vi "Stop Test.vi"(8 "ErrorIn":errorcluster, 11 "VISAIn":refnum<visa-resource-name>) -> (0 "ErrorOut":errorcluster, 2 "Data":string, 3 "VISAOut":refnum<visa-resource-name>)   [LabVIEW 2017, in "I28Drivers.lvlib"]
uses:
  I28Drivers.lvlib
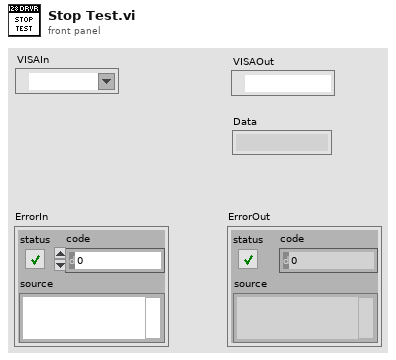
[diagram p1: front panel]
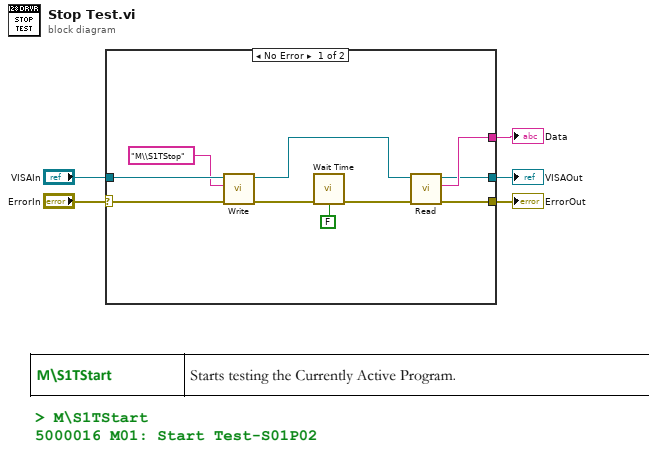
[diagram p0: block diagram]
diagram:
  n1 = case shown="No Error" "ErrorIn" {
    selector: "ErrorIn" -> [w15 w16]
    tunnel: "VISAIn" -> [w14 w17]
    tunnel: [w12 _] -> w3
    tunnel: [w11 w17] -> w1
    tunnel: [w10 w16] -> w2
    frame No Error {
      n2 = call "Write.vi"("ErrorIn"=w15, "Command"="M\\S1TStop", "VISAIn"=w14) -> ("ErrorOut"=w8:errorcluster, "VISAOut"=w9:refnum<visa-resource-name>)  [unwired: 7 in]
      n3 = call "Wait Time.vi"("error in"=w8, "Set Time"=FALSE) -> ("error out"=w7:errorcluster)  [unwired: 13 in]
      n4 = call "Read.vi"("ErrorIn"=w7, "VISAIn"=w9) -> ("ErrorOut"=w10:errorcluster, "Data"=w12:string, "VISAOut"=w11:refnum<visa-resource-name>)  [unwired: 7 in]
    }
    frame Error {
    }
  }
  "ErrorOut" <- w2
  "Data" <- w3
  "VISAOut" <- w1
